vi "ArrayFormula.vi"() -> ()   [LabVIEW 2014]
uses:
  <vilib>/gmath/NI_Gmath.lvlib
panel:
  out "Parsed Formula":cluster{"Table":i32[][], "Y Values":dbl[]} {"Y Values" format="%.2f"}
  out "Tree formula":T1(array[cluster])
  # "[0 1]\n[0+1]\n[W0+W1]"
  # "operator"
  # "register1"
  # "register2"
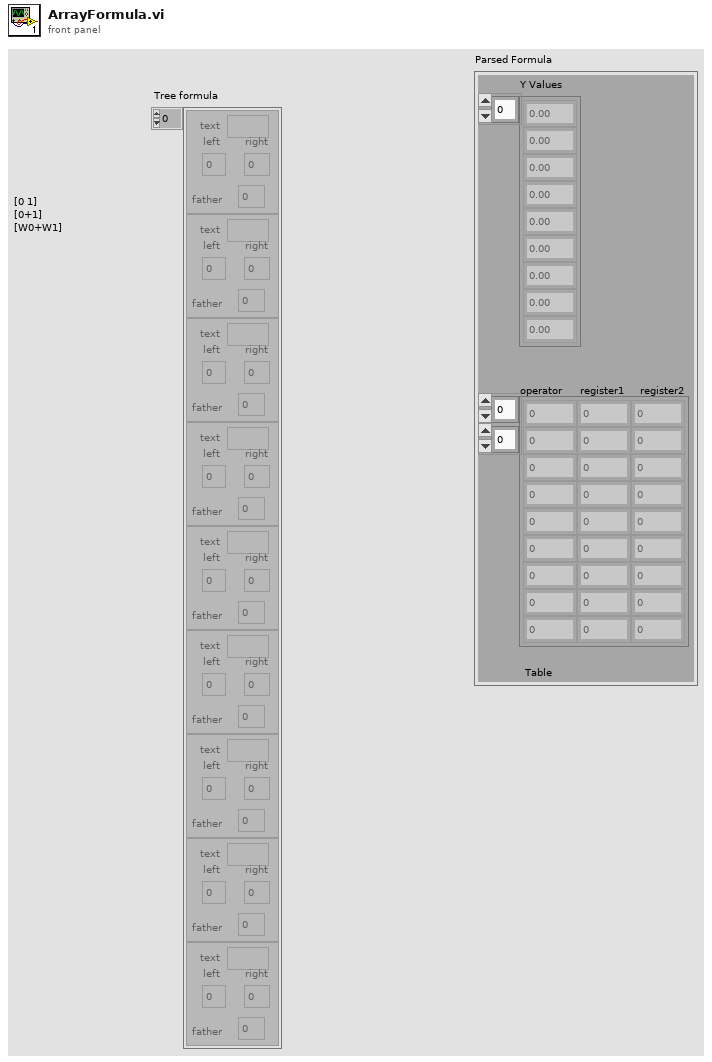
[diagram p1: front panel]
types:
  T1 = cluster{"text":string, "left":i32, "right":i32, "father":i32}[]
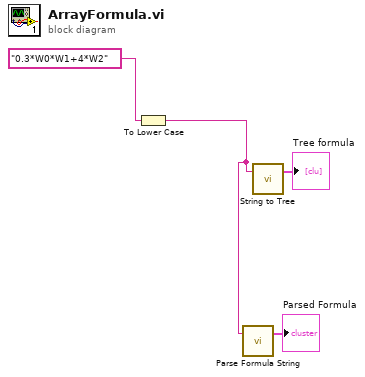
[diagram p0: block diagram]
diagram:
  n1 = To Lower Case(string="0.3*W0*W1+4*W2" ("formula")) -> (all lower case string=w1:string)
  n2 = call <vilib>:"Parse Formula String.vi"("formula"=w1) -> ("Parsed Formula"=→"Parsed Formula":cluster{"Table":i32[][], "Y Values":dbl[]})  [unwired: 1 in, 1 out]
  n3 = call <vilib>:"String to Tree.VI"("user formula"=w1) -> ("Tree formula"=→"Tree formula":T1)  [unwired: 1 in, 1 out]
